vi "Delta_Array.vi"(5 "variableArray":string[][](array[string]), 6 "previousVar":string, 7 "index":i32, 8 "inputArray":dbl[](array[numeric]), 9 "deltaArray":dbl[][](array[numeric]), 10 "currentValue":dbl) -> (0 "outputText":string, 1 "outputArray":dbl[](array[numeric]), 3 "triggerEvent":bool)   [LabVIEW 2019]
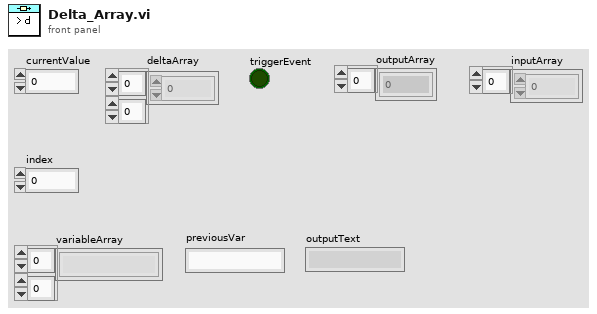
[diagram p1: front panel]
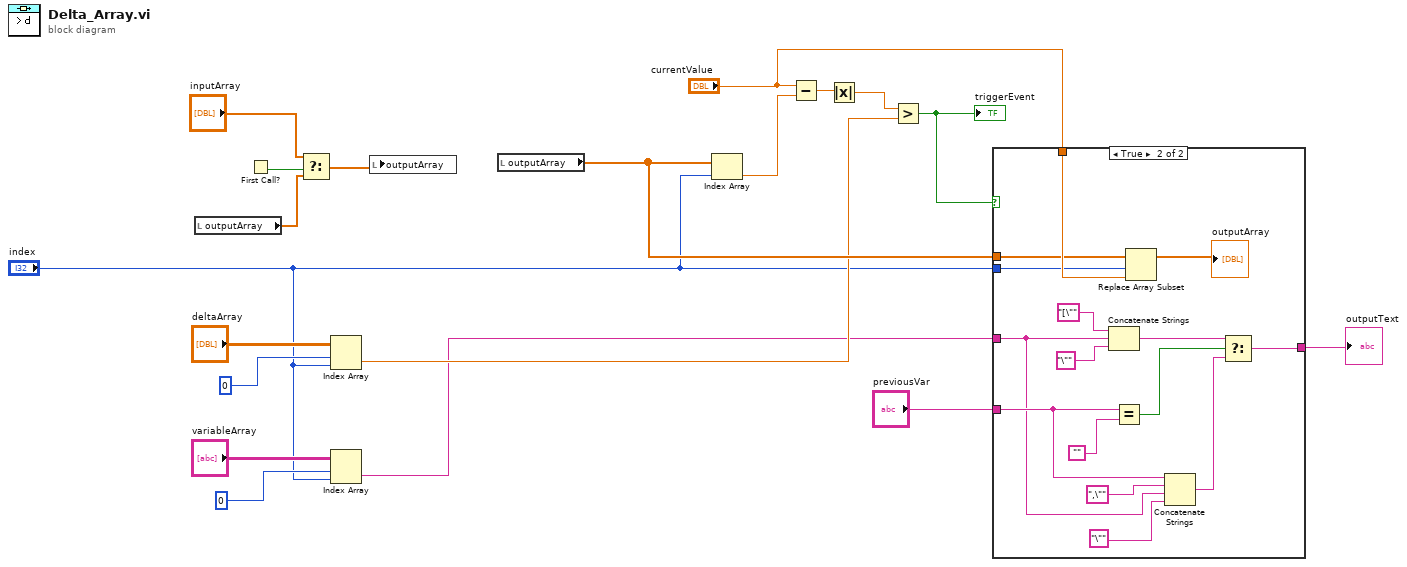
[diagram p0: block diagram]
diagram:
  n1 = local read "outputArray"() -> (w15:dbl[])
  n2 = First Call?() -> (First Call?: T/F=w14:bool)
  n3 = Select(t="inputArray", s=w14, f=w15) -> (s? t:f=w13:dbl[])
  n4 = Index Array(array="deltaArray", index (row)=0, index (col)="index") -> (element=w6:dbl)
  n5 = Index Array(array="variableArray", index (row)=0, index (col)="index") -> (element=w2:string)
  n6 = local write "outputArray"(w13) -> ()
  n7 = local read "outputArray"() -> (w12:dbl[])
  n8 = Index Array(array=w12, index="index") -> (element=w16:dbl)
  n9 = Subtract(x="currentValue", y=w16) -> (x-y=w17:dbl)
  n10 = Absolute Value(x=w17) -> (abs(x)=w18:dbl)
  n11 = Greater?(x=w18, y=w6) -> (0:w11:bool)
  "triggerEvent" <- w11
  n12 = case shown="True" w11 {
    tunnel: "currentValue" -> [_ w35]
    tunnel: "index" -> [_ w34]
    tunnel: w12 -> [_ w32]
    tunnel: w2 -> [_ w21]
    tunnel: "previousVar" -> [w20 w22]
    tunnel: [w20 w27] -> w9
    frame False {
    }
    frame True {
      n13 = Concatenate Strings("[\"", w21, "\"") -> (w26:string)
      n14 = Equal?(x=w22, y="") -> (x = y?=w30:bool)
      n15 = Replace Array Subset(array=w32, new element=w35, index=w34) -> (→"outputArray":dbl[])
      n16 = Concatenate Strings(w22, ",\"", w21, "\"") -> (w28:string)
      n17 = Select(t=w26, s=w30, f=w28) -> (s? t:f=w27:string)
    }
  }
  "outputText" <- w9
